vi "replace plot - plot ref - V2.vi"(0 "Plot ref in":refnum<vi>, 1 "Array X IN":dbl[](array[numeric]), 2 "Array Y IN":dbl[](array[numeric]), 3 "text":string="x", 5 "plot index":i32, 6 "cursor action":T2=enum."write", 7 "label":enum16{"hide", "show x", "show y", "show (x,y)"}(ring), 12 "Color Box":u32(colorbox)=327424, 13 "cursor state":T3=enum."boring") -> (14 "Plot ref out":refnum<vi>, 15 "Array X":dbl[](array[numeric]), 16 "Array Y":dbl[](array[numeric]), 19 "2Dwindow bounds out":T1={"min y"=0.0021014740628288917, "max x"=44850.89441339177, "min x"=2.5658109925320947, "max y"=17480.201988350764} {"max y" format="%#9_9f"; "min x" format="%#9_9f"; "max x" format="%#9_9f"})   [LabVIEW 2021]
uses:
  cursor sate.ctl
  cursor action.ctl
  2Dwindow-bounds.ctl
  stack action -- control.ctl
  range multiplier action.ctl
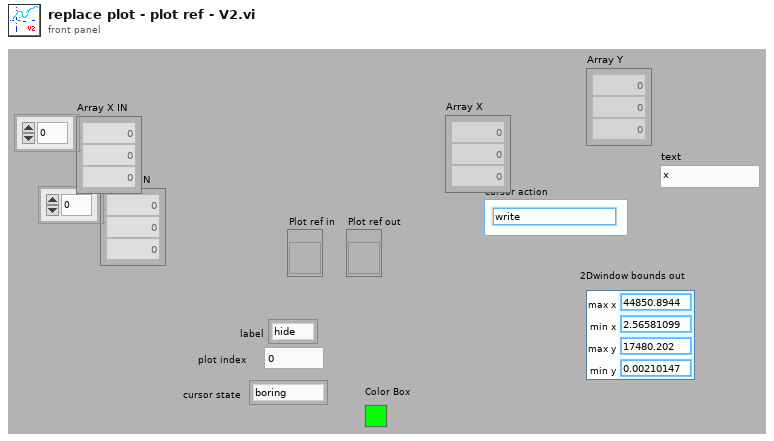
[diagram p1: front panel]
types:
  T1 = typedef "2Dwindow-bounds.ctl" = cluster{"min y":dbl, "max x":dbl, "min x":dbl, "max y":dbl}
  T2 = typedef "cursor action.ctl" = enum16{"range", "read", "write", "check", "zoom out", "smart zoom out", "zoom to aspect ratio 1", "zoom to win", "zoom out 20%", "zoom in 20%", "-empty", "smart zoom out&aspect", "move range left 20%", "move range right 20%", "move range up 20%", "move range down 20%", "zoom to X win", "zoom to Y win", "zoom out X", "zoom out Y", "zoom in X", "zoom in Y", "check plot scale", "set plot color", "set Xlabel", "set Ylabel", "set cursor color"}
  T3 = typedef "cursor sate.ctl" = enum16{"normal", "alert", "fuzzy", "interesting", "boring", "colored"}
  T4 = typedef "stack action -- control.ctl" = enum16{"push", "pop", "check", "init"}
  T5 = typedef "range multiplier action.ctl" = enum16{"shift", "zoom", "check"}
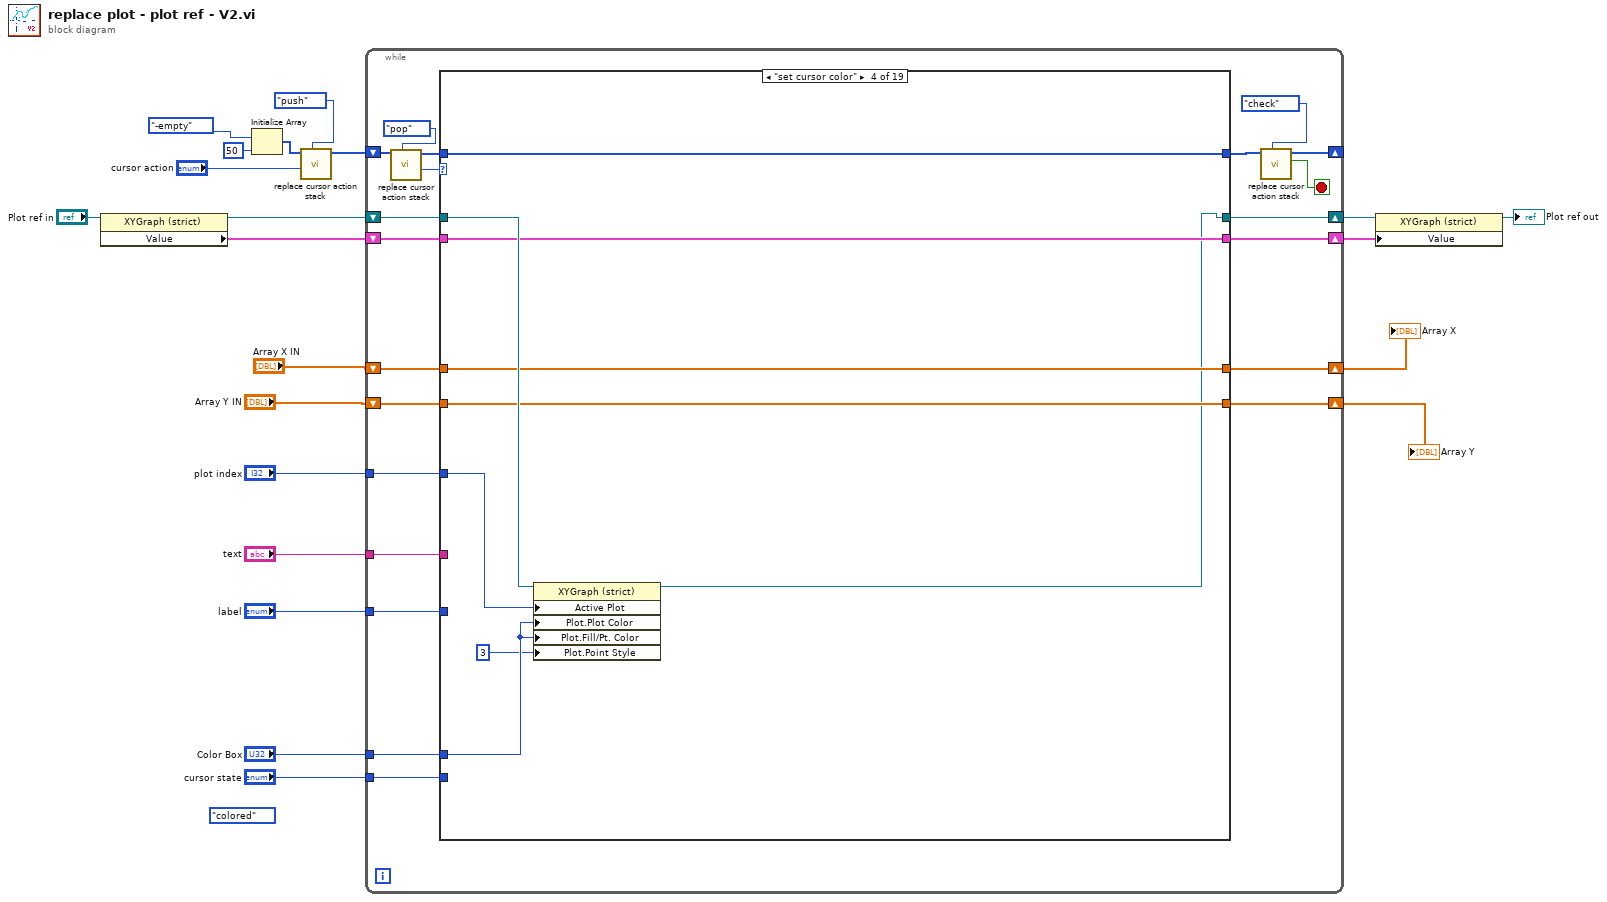
[diagram p0: block diagram]
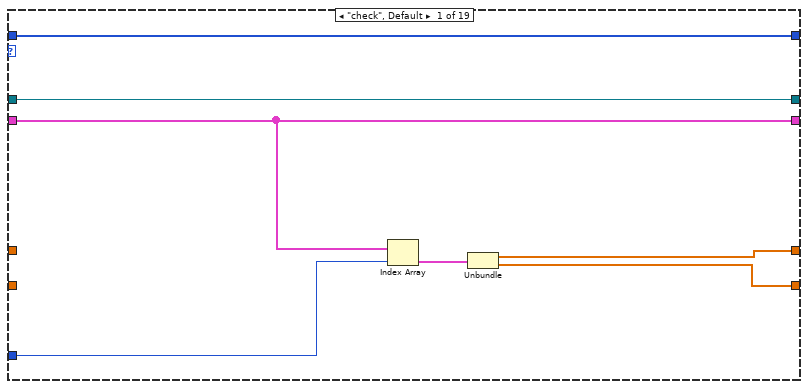
[diagram p2: hidden frame]
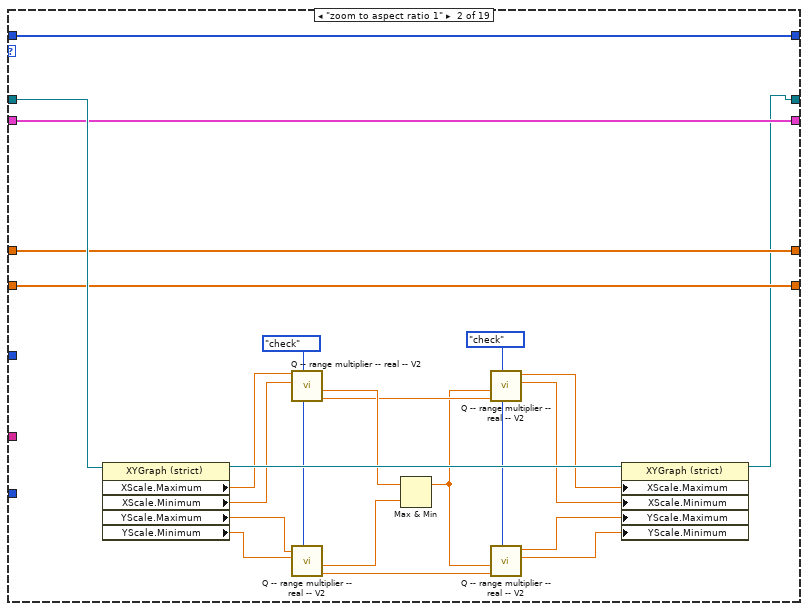
[diagram p3: hidden frame]
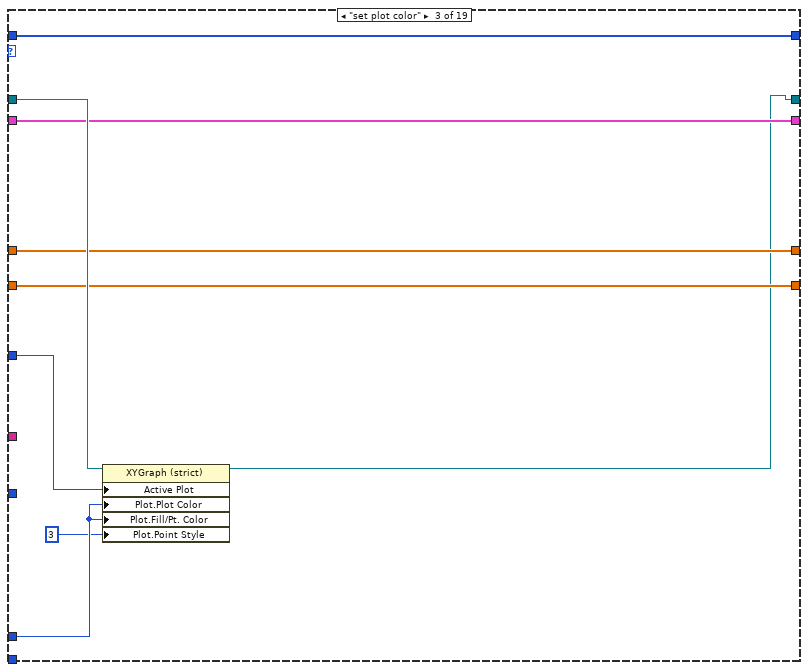
[diagram p4: hidden frame]
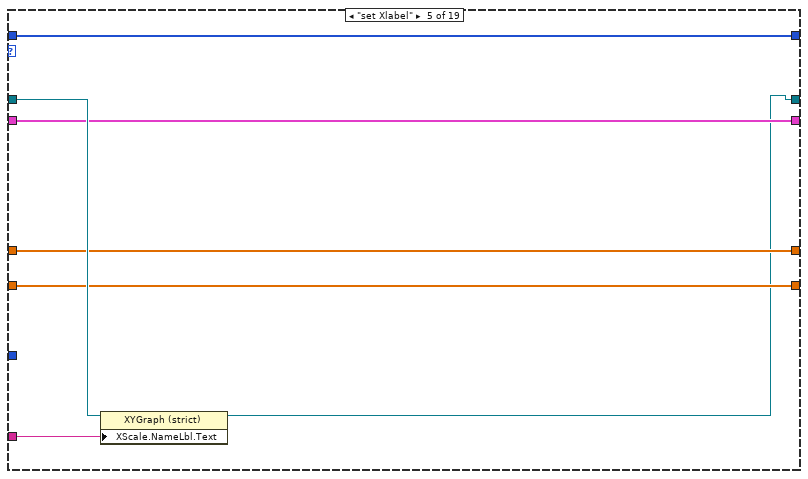
[diagram p5: hidden frame]
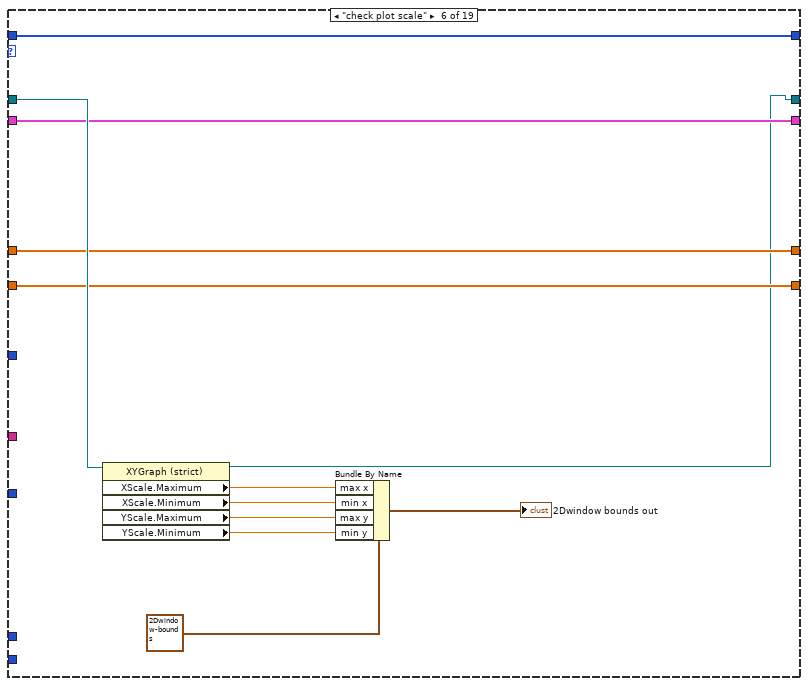
[diagram p6: hidden frame]
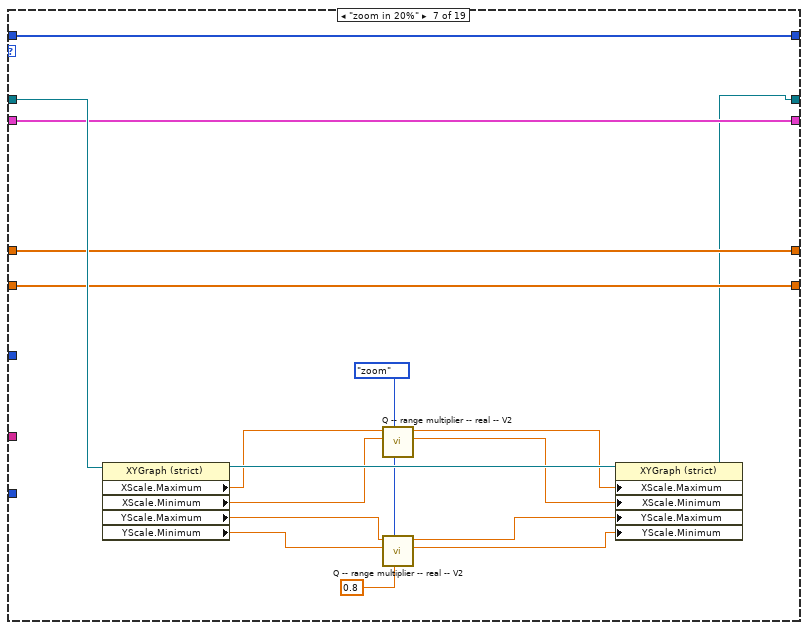
[diagram p7: hidden frame]
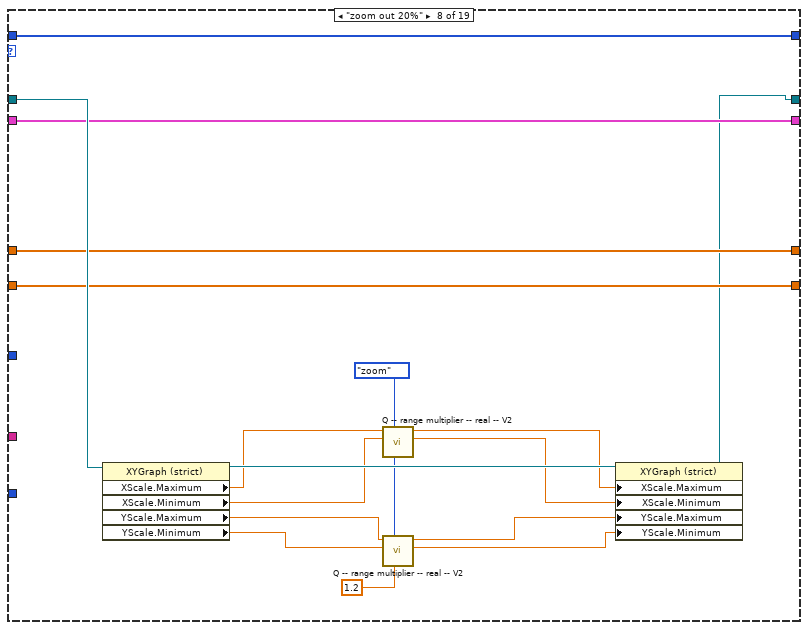
[diagram p8: hidden frame]
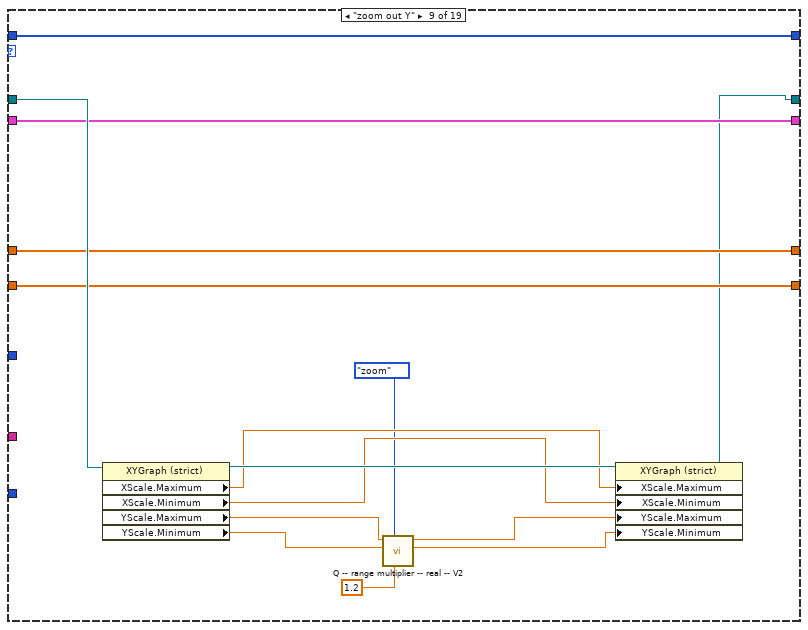
[diagram p9: hidden frame]
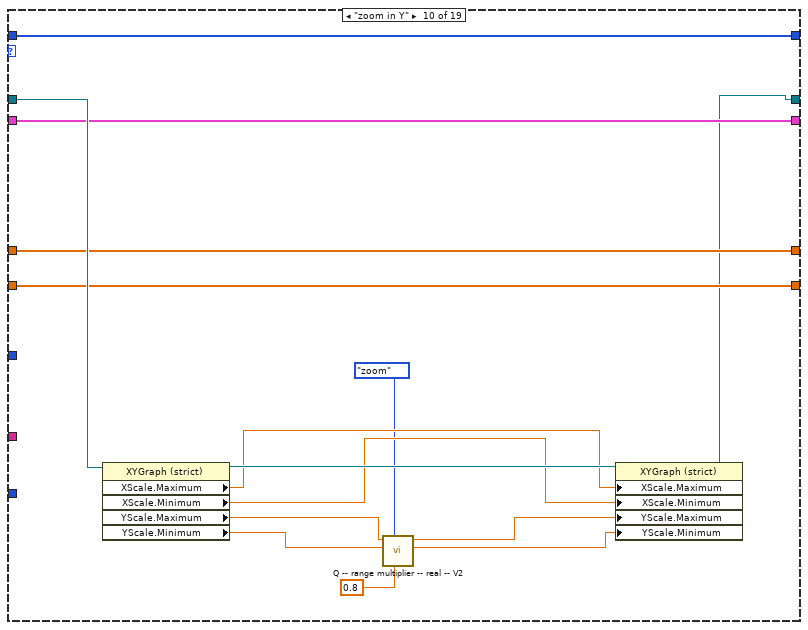
[diagram p10: hidden frame]
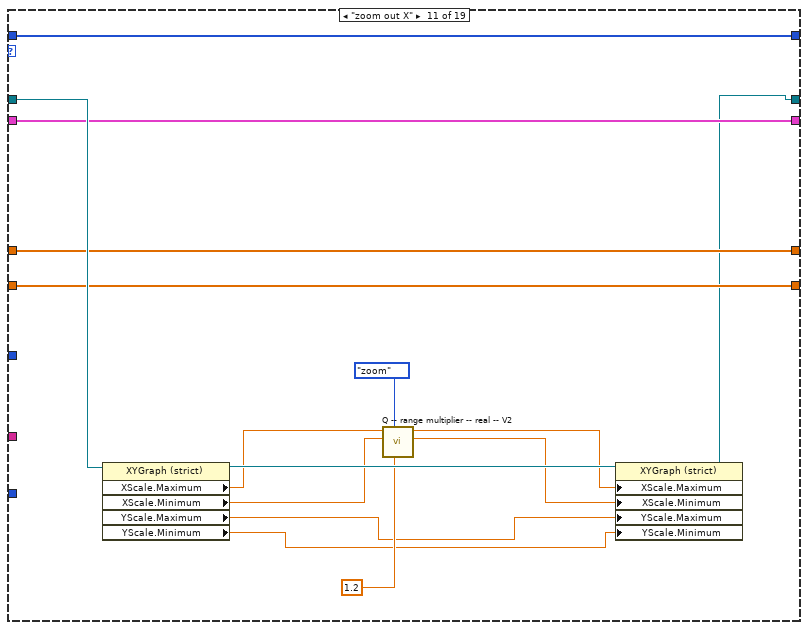
[diagram p11: hidden frame]
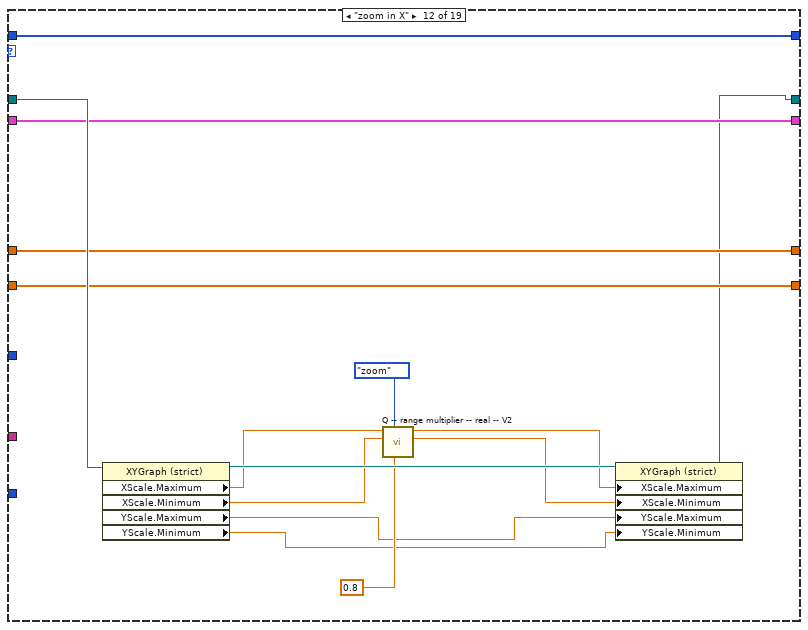
[diagram p12: hidden frame]
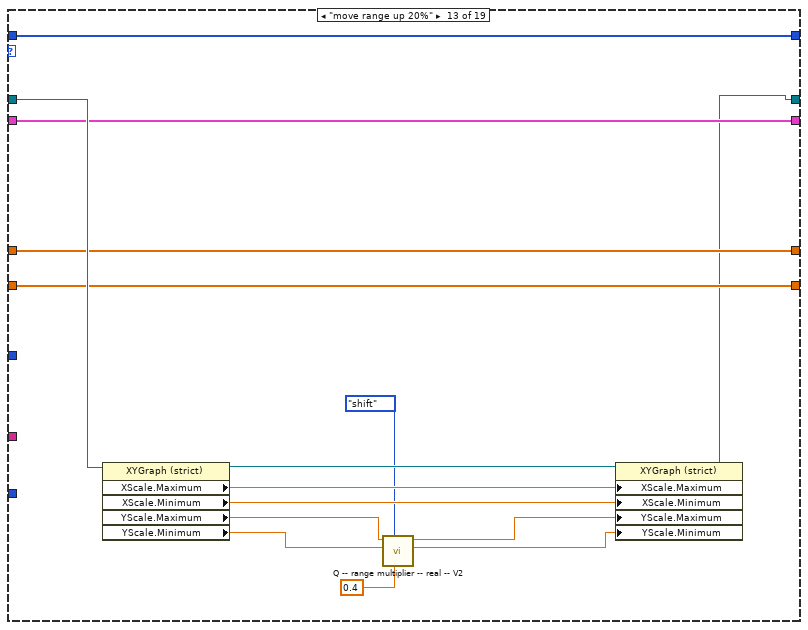
[diagram p13: hidden frame]
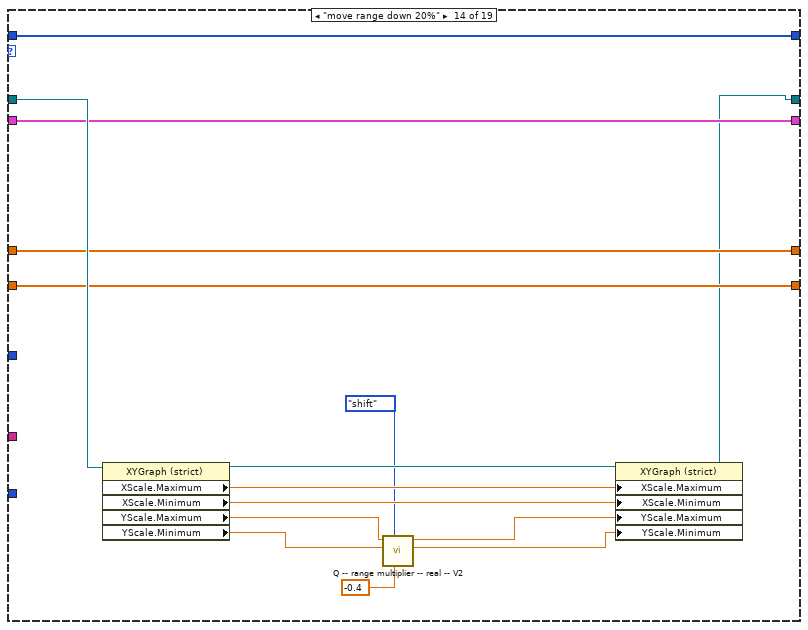
[diagram p14: hidden frame]
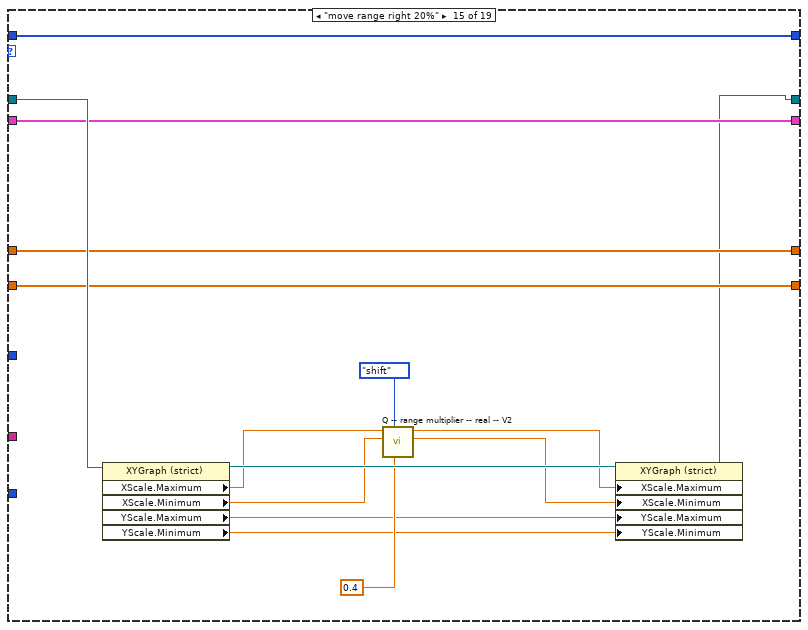
[diagram p15: hidden frame]
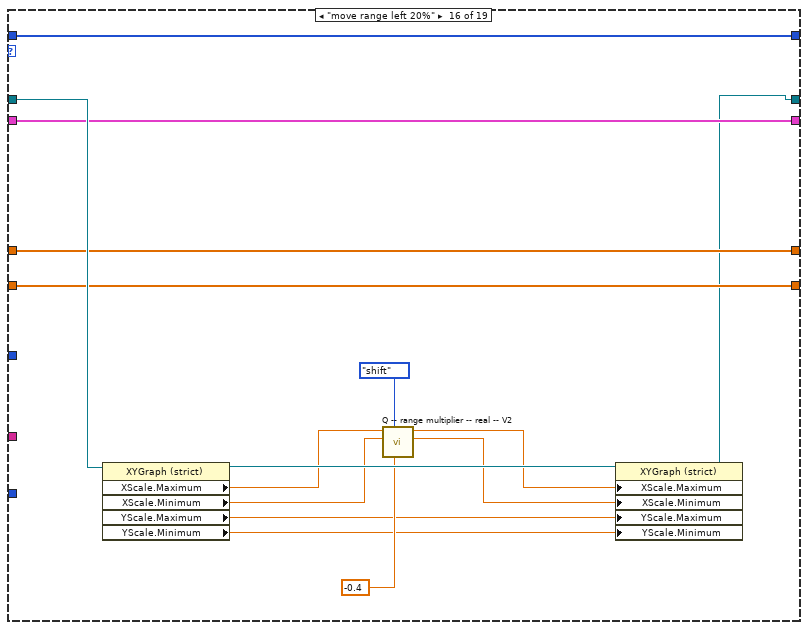
[diagram p16: hidden frame]
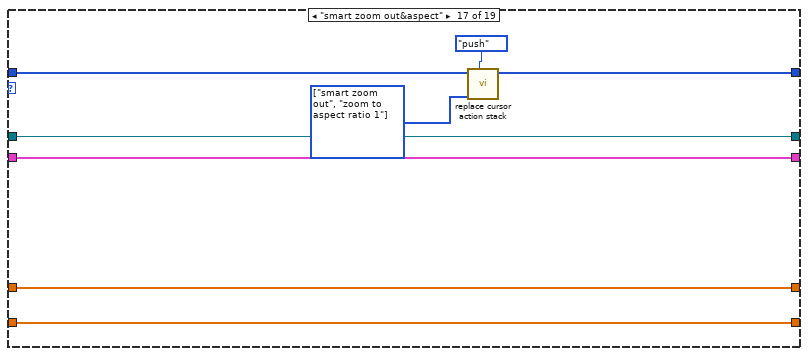
[diagram p17: hidden frame]
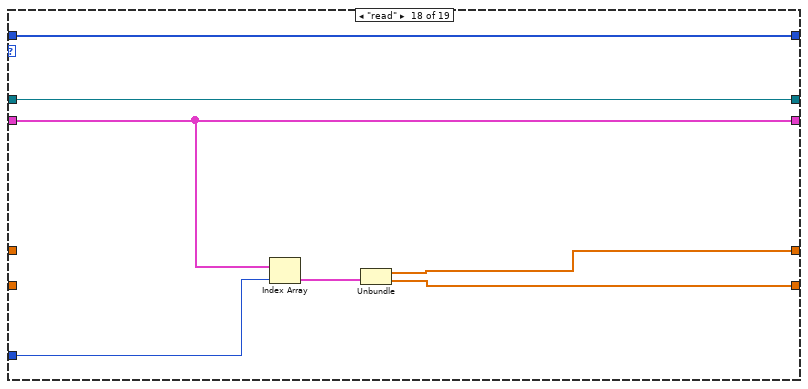
[diagram p18: hidden frame]
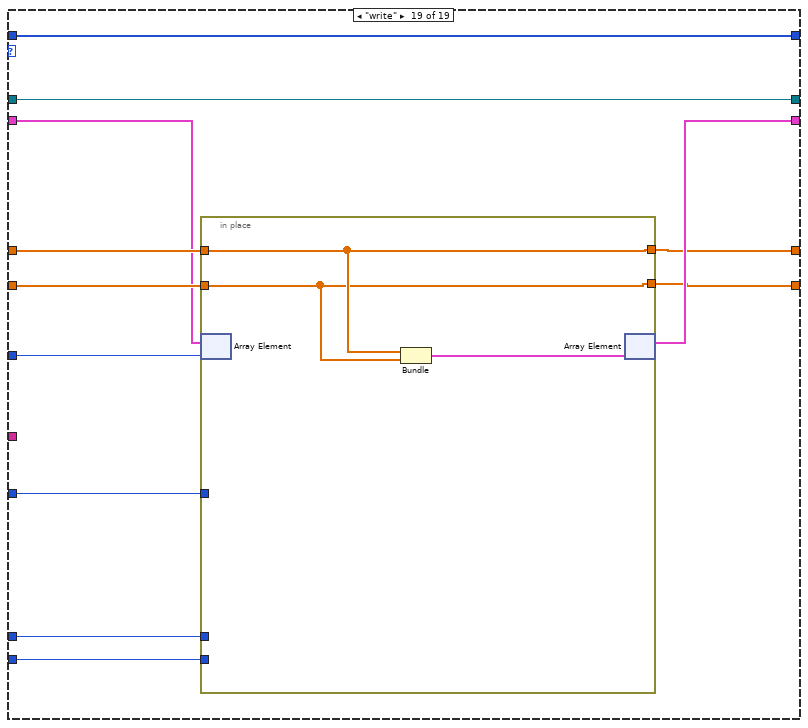
[diagram p19: hidden frame]
diagram:
  (unwired) cursor_sate."colored" ("cursor state")
  n1 = property on="Property Node" class="XYGraph (strict)"(reference="Plot ref in") -> (reference out=w13:refnum<vi>, "Value"=w20:cluster{dbl[], dbl[]}[])  [unwired: 1 in, 1 out]
  n2 = Initialize Array(cursor_action."-empty" ("cursor action"), 50 ("dimension size")) -> (w9:T2[])
  n3 = call "replace cursor action stack.vi"("stack action"=stack_action_--_control."push", "cursor action"="cursor action", "command stack In"=w9) -> ("command stack Out"=w6:T2[])  [unwired: 6 in, 2 out]
  n4 = while {
    tunnel: "plot index" -> [w42]
    tunnel: "label" -> [w38]
    tunnel: "Color Box" -> [w37]
    tunnel: "cursor state" -> [w36]
    shift-right: [w33] -> w12
    shift-left: w20 -> [w39]
    shift-right: [w35] -> w14
    shift-left: w13 -> [w34]
    shift-right: [w28] -> _
    shift-left: w6 -> [w32]
    shift-right: [w25] -> w4
    shift-left: "Array Y IN" -> [w41]
    shift-right: [w24] -> w5
    shift-left: "Array X IN" -> [w40]
    tunnel: "text" -> [w22]
    stop <- w29 stop-if-true
    n5 = call "replace cursor action stack.vi"("stack action"=stack_action_--_control."pop", "command stack In"=w32) -> ("cursor action Out"=w30:T2, "command stack Out"=w26:T2[])  [unwired: 7 in, 1 out]
    n6 = case shown="\"set cursor color\"" w30 {
      tunnel: w42 -> [w47 _ w75 w84 _ _ _ _ _ _ _ _ _ _ _ _ _ w277 w285]
      tunnel: w39 -> [w48 w69 w79 w88 w95 w107 w123 w140 w155 w170 w185 w200 w215 w230 w245 w260 w263 w276 w287]
      tunnel: w41 -> [_ w67 w77 w86 w93 w105 w121 w138 w153 w168 w183 w198 w213 w228 w243 w258 w265 _ w288]
      tunnel: w40 -> [_ w68 w78 w87 w94 w106 w122 w139 w154 w169 w184 w199 w214 w229 w244 w259 w266 _ w289]
      tunnel: [w44 w68 w78 w87 w94 w106 w122 w139 w154 w169 w184 w199 w214 w229 w244 w259 w266 w272 w284] -> w24
      tunnel: [w43 w67 w77 w86 w93 w105 w121 w138 w153 w168 w183 w198 w213 w228 w243 w258 w265 w271 w283] -> w25
      tunnel: w38 -> [_ _ _ _ _ _ _ _ _ _ _ _ _ _ _ _ _ _ w282]
      tunnel: w37 -> [_ _ w73 w82 _ _ _ _ _ _ _ _ _ _ _ _ _ _ w281]
      tunnel: w36 -> [_ _ _ _ _ _ _ _ _ _ _ _ _ _ _ _ _ _ w280]
      tunnel: [w49 w65 w74 w83 w91 w103 w119 w136 w151 w166 w181 w196 w211 w226 w241 w256 w264 w275 w279] -> w35
      tunnel: w34 -> [w49 w70 w80 w89 w96 w108 w124 w141 w156 w171 w186 w201 w216 w231 w246 w261 w264 w275 w279]
      tunnel: [w48 w69 w79 w88 w95 w107 w123 w140 w155 w170 w185 w200 w215 w230 w245 w260 w263 w276 w286] -> w33
      tunnel: [w46 w66 w76 w85 w92 w104 w120 w137 w152 w167 w182 w197 w212 w227 w242 w257 w268 w274 w278] -> w27
      tunnel: w26 -> [w46 w66 w76 w85 w92 w104 w120 w137 w152 w167 w182 w197 w212 w227 w242 w257 w269 w274 w278]
      tunnel: w22 -> [_ _ _ _ w90 _ _ _ _ _ _ _ _ _ _ _ _ _ _]
      frame "check", Default {
        n7 = Index Array(array=w48, index=w47) -> (element=w45:cluster{dbl[], dbl[]})
        n8 = Unbundle(w45) -> (w44:dbl[], w43:dbl[])
      }
      frame "zoom to aspect ratio 1" {
        w54 = range_multiplier_action."check" ("rage multiplier action")
        w60 = range_multiplier_action."check" ("rage multiplier action")
        n9 = property on="Property Node" class="XYGraph (strict)"(reference=w70) -> (reference out=w71:refnum<vi>, "XScale.Maximum"=w64:dbl, "XScale.Minimum"=w63:dbl, "YScale.Maximum"=w62:dbl, "YScale.Minimum"=w61:dbl)  [unwired: 1 in, 1 out]
        n10 = call "Q -- range multiplier -- real -- V2.vi"("rage multiplier action"=w60, "lower"=w63, "upper"=w64) -> ("center OUT"=w57:dbl, "window OUT"=w59:dbl)  [unwired: 5 in, 2 out]
        n11 = call "Q -- range multiplier -- real -- V2.vi"("rage multiplier action"=w60, "lower"=w61, "upper"=w62) -> ("center OUT"=w56:dbl, "window OUT"=w58:dbl)  [unwired: 5 in, 2 out]
        n12 = Max & Min(x=w59, y=w58) -> (max(x,y)=w55:dbl)  [unwired: 1 out]
        n13 = call "Q -- range multiplier -- real -- V2.vi"("rage multiplier action"=w54, "center"=w57, "window"=w55) -> ("lower OUT"=w50:dbl, "upper OUT"=w51:dbl)  [unwired: 5 in, 2 out]
        n14 = call "Q -- range multiplier -- real -- V2.vi"("rage multiplier action"=w54, "center"=w56, "window"=w55) -> ("lower OUT"=w52:dbl, "upper OUT"=w53:dbl)  [unwired: 5 in, 2 out]
        n15 = property on="Property Node" class="XYGraph (strict)"(reference=w71, "XScale.Maximum"=w51, "XScale.Minimum"=w50, "YScale.Maximum"=w53, "YScale.Minimum"=w52) -> (reference out=w65:refnum<vi>)  [unwired: 1 in, 1 out]
      }
      frame "set plot color" {
        n16 = property on="Property Node" class="XYGraph (strict)"(reference=w80, "Active Plot"=w75, "Plot.Plot Color"=w73, "Plot.Fill/Pt. Color"=w73, "Plot.Point Style"=u8 3) -> (reference out=w74:refnum<vi>)  [unwired: 1 in, 1 out]
      }
      frame "set cursor color" {
        n17 = property on="Property Node" class="XYGraph (strict)"(reference=w89, "Active Plot"=w84, "Plot.Plot Color"=w82, "Plot.Fill/Pt. Color"=w82, "Plot.Point Style"=u8 3) -> (reference out=w83:refnum<vi>)  [unwired: 1 in, 1 out]
      }
      frame "set Xlabel" {
        n18 = property on="Property Node" class="XYGraph (strict)"(reference=w96, "XScale.NameLbl.Text"=w90) -> (reference out=w91:refnum<vi>)  [unwired: 1 in, 1 out]
      }
      frame "check plot scale" {
        n19 = property on="Property Node" class="XYGraph (strict)"(reference=w108) -> (reference out=w103:refnum<vi>, "XScale.Maximum"=w101:dbl, "XScale.Minimum"=w100:dbl, "YScale.Maximum"=w99:dbl, "YScale.Minimum"=w98:dbl)  [unwired: 1 in, 1 out]
        n20 = Bundle By Name(cluster=T1 {"min y"=0.0021014740628288917, "max x"=44850.89441339177, "min x"=2.5658109925320947, "max y"=17480.201988350764} ("2Dwindow bounds out"), "max x"=w101, "min x"=w100, "max y"=w99, "min y"=w98) -> (→"2Dwindow bounds out":T1)
      }
      frame "zoom in 20%" {
        w110 = range_multiplier_action."zoom" ("rage multiplier action")
        w109 = 0.8
        n21 = property on="Property Node" class="XYGraph (strict)"(reference=w124) -> (reference out=w125:refnum<vi>, "XScale.Maximum"=w118:dbl, "XScale.Minimum"=w117:dbl, "YScale.Maximum"=w114:dbl, "YScale.Minimum"=w113:dbl)  [unwired: 1 in, 1 out]
        n22 = call "Q -- range multiplier -- real -- V2.vi"("factor"=w109, "rage multiplier action"=w110, "lower"=w117, "upper"=w118) -> ("lower OUT"=w115:dbl, "upper OUT"=w116:dbl)  [unwired: 4 in, 2 out]
        n23 = call "Q -- range multiplier -- real -- V2.vi"("factor"=w109, "rage multiplier action"=w110, "lower"=w113, "upper"=w114) -> ("lower OUT"=w111:dbl, "upper OUT"=w112:dbl)  [unwired: 4 in, 2 out]
        n24 = property on="Property Node" class="XYGraph (strict)"(reference=w125, "XScale.Maximum"=w116, "XScale.Minimum"=w115, "YScale.Maximum"=w112, "YScale.Minimum"=w111) -> (reference out=w119:refnum<vi>)  [unwired: 1 in, 1 out]
      }
      frame "zoom out 20%" {
        w127 = range_multiplier_action."zoom" ("rage multiplier action")
        w126 = 1.2
        n25 = property on="Property Node" class="XYGraph (strict)"(reference=w141) -> (reference out=w142:refnum<vi>, "XScale.Maximum"=w135:dbl, "XScale.Minimum"=w134:dbl, "YScale.Maximum"=w131:dbl, "YScale.Minimum"=w130:dbl)  [unwired: 1 in, 1 out]
        n26 = call "Q -- range multiplier -- real -- V2.vi"("factor"=w126, "rage multiplier action"=w127, "lower"=w134, "upper"=w135) -> ("lower OUT"=w132:dbl, "upper OUT"=w133:dbl)  [unwired: 4 in, 2 out]
        n27 = call "Q -- range multiplier -- real -- V2.vi"("factor"=w126, "rage multiplier action"=w127, "lower"=w130, "upper"=w131) -> ("lower OUT"=w128:dbl, "upper OUT"=w129:dbl)  [unwired: 4 in, 2 out]
        n28 = property on="Property Node" class="XYGraph (strict)"(reference=w142, "XScale.Maximum"=w133, "XScale.Minimum"=w132, "YScale.Maximum"=w129, "YScale.Minimum"=w128) -> (reference out=w136:refnum<vi>)  [unwired: 1 in, 1 out]
      }
      frame "zoom out Y" {
        n29 = property on="Property Node" class="XYGraph (strict)"(reference=w156) -> (reference out=w157:refnum<vi>, "XScale.Maximum"=w145:dbl, "XScale.Minimum"=w144:dbl, "YScale.Maximum"=w150:dbl, "YScale.Minimum"=w149:dbl)  [unwired: 1 in, 1 out]
        n30 = call "Q -- range multiplier -- real -- V2.vi"("factor"=1.2, "rage multiplier action"=range_multiplier_action."zoom", "lower"=w149, "upper"=w150) -> ("lower OUT"=w147:dbl, "upper OUT"=w148:dbl)  [unwired: 4 in, 2 out]
        n31 = property on="Property Node" class="XYGraph (strict)"(reference=w157, "XScale.Maximum"=w145, "XScale.Minimum"=w144, "YScale.Maximum"=w148, "YScale.Minimum"=w147) -> (reference out=w151:refnum<vi>)  [unwired: 1 in, 1 out]
      }
      frame "zoom in Y" {
        n32 = property on="Property Node" class="XYGraph (strict)"(reference=w171) -> (reference out=w172:refnum<vi>, "XScale.Maximum"=w160:dbl, "XScale.Minimum"=w159:dbl, "YScale.Maximum"=w165:dbl, "YScale.Minimum"=w164:dbl)  [unwired: 1 in, 1 out]
        n33 = call "Q -- range multiplier -- real -- V2.vi"("factor"=0.8, "rage multiplier action"=range_multiplier_action."zoom", "lower"=w164, "upper"=w165) -> ("lower OUT"=w162:dbl, "upper OUT"=w163:dbl)  [unwired: 4 in, 2 out]
        n34 = property on="Property Node" class="XYGraph (strict)"(reference=w172, "XScale.Maximum"=w160, "XScale.Minimum"=w159, "YScale.Maximum"=w163, "YScale.Minimum"=w162) -> (reference out=w166:refnum<vi>)  [unwired: 1 in, 1 out]
      }
      frame "zoom out X" {
        n35 = property on="Property Node" class="XYGraph (strict)"(reference=w186) -> (reference out=w187:refnum<vi>, "XScale.Maximum"=w180:dbl, "XScale.Minimum"=w179:dbl, "YScale.Maximum"=w174:dbl, "YScale.Minimum"=w173:dbl)  [unwired: 1 in, 1 out]
        n36 = call "Q -- range multiplier -- real -- V2.vi"("factor"=1.2, "rage multiplier action"=range_multiplier_action."zoom", "lower"=w179, "upper"=w180) -> ("lower OUT"=w177:dbl, "upper OUT"=w178:dbl)  [unwired: 4 in, 2 out]
        n37 = property on="Property Node" class="XYGraph (strict)"(reference=w187, "XScale.Maximum"=w178, "XScale.Minimum"=w177, "YScale.Maximum"=w174, "YScale.Minimum"=w173) -> (reference out=w181:refnum<vi>)  [unwired: 1 in, 1 out]
      }
      frame "zoom in X" {
        n38 = property on="Property Node" class="XYGraph (strict)"(reference=w201) -> (reference out=w202:refnum<vi>, "XScale.Maximum"=w195:dbl, "XScale.Minimum"=w194:dbl, "YScale.Maximum"=w189:dbl, "YScale.Minimum"=w188:dbl)  [unwired: 1 in, 1 out]
        n39 = call "Q -- range multiplier -- real -- V2.vi"("factor"=0.8, "rage multiplier action"=range_multiplier_action."zoom", "lower"=w194, "upper"=w195) -> ("lower OUT"=w192:dbl, "upper OUT"=w193:dbl)  [unwired: 4 in, 2 out]
        n40 = property on="Property Node" class="XYGraph (strict)"(reference=w202, "XScale.Maximum"=w193, "XScale.Minimum"=w192, "YScale.Maximum"=w189, "YScale.Minimum"=w188) -> (reference out=w196:refnum<vi>)  [unwired: 1 in, 1 out]
      }
      frame "move range up 20%" {
        n41 = property on="Property Node" class="XYGraph (strict)"(reference=w216) -> (reference out=w217:refnum<vi>, "XScale.Maximum"=w204:dbl, "XScale.Minimum"=w205:dbl, "YScale.Maximum"=w210:dbl, "YScale.Minimum"=w209:dbl)  [unwired: 1 in, 1 out]
        n42 = call "Q -- range multiplier -- real -- V2.vi"("factor"=0.4, "rage multiplier action"=range_multiplier_action."shift", "lower"=w209, "upper"=w210) -> ("lower OUT"=w207:dbl, "upper OUT"=w208:dbl)  [unwired: 4 in, 2 out]
        n43 = property on="Property Node" class="XYGraph (strict)"(reference=w217, "XScale.Maximum"=w204, "XScale.Minimum"=w205, "YScale.Maximum"=w208, "YScale.Minimum"=w207) -> (reference out=w211:refnum<vi>)  [unwired: 1 in, 1 out]
      }
      frame "move range down 20%" {
        n44 = property on="Property Node" class="XYGraph (strict)"(reference=w231) -> (reference out=w232:refnum<vi>, "XScale.Maximum"=w219:dbl, "XScale.Minimum"=w220:dbl, "YScale.Maximum"=w225:dbl, "YScale.Minimum"=w224:dbl)  [unwired: 1 in, 1 out]
        n45 = call "Q -- range multiplier -- real -- V2.vi"("factor"=-0.4, "rage multiplier action"=range_multiplier_action."shift", "lower"=w224, "upper"=w225) -> ("lower OUT"=w222:dbl, "upper OUT"=w223:dbl)  [unwired: 4 in, 2 out]
        n46 = property on="Property Node" class="XYGraph (strict)"(reference=w232, "XScale.Maximum"=w219, "XScale.Minimum"=w220, "YScale.Maximum"=w223, "YScale.Minimum"=w222) -> (reference out=w226:refnum<vi>)  [unwired: 1 in, 1 out]
      }
      frame "move range right 20%" {
        n47 = property on="Property Node" class="XYGraph (strict)"(reference=w246) -> (reference out=w247:refnum<vi>, "XScale.Maximum"=w240:dbl, "XScale.Minimum"=w239:dbl, "YScale.Maximum"=w234:dbl, "YScale.Minimum"=w233:dbl)  [unwired: 1 in, 1 out]
        n48 = call "Q -- range multiplier -- real -- V2.vi"("factor"=0.4, "rage multiplier action"=range_multiplier_action."shift", "lower"=w239, "upper"=w240) -> ("lower OUT"=w237:dbl, "upper OUT"=w238:dbl)  [unwired: 4 in, 2 out]
        n49 = property on="Property Node" class="XYGraph (strict)"(reference=w247, "XScale.Maximum"=w238, "XScale.Minimum"=w237, "YScale.Maximum"=w234, "YScale.Minimum"=w233) -> (reference out=w241:refnum<vi>)  [unwired: 1 in, 1 out]
      }
      frame "move range left 20%" {
        n50 = property on="Property Node" class="XYGraph (strict)"(reference=w261) -> (reference out=w262:refnum<vi>, "XScale.Maximum"=w255:dbl, "XScale.Minimum"=w254:dbl, "YScale.Maximum"=w249:dbl, "YScale.Minimum"=w248:dbl)  [unwired: 1 in, 1 out]
        n51 = call "Q -- range multiplier -- real -- V2.vi"("factor"=-0.4, "rage multiplier action"=range_multiplier_action."shift", "lower"=w254, "upper"=w255) -> ("lower OUT"=w252:dbl, "upper OUT"=w253:dbl)  [unwired: 4 in, 2 out]
        n52 = property on="Property Node" class="XYGraph (strict)"(reference=w262, "XScale.Maximum"=w253, "XScale.Minimum"=w252, "YScale.Maximum"=w249, "YScale.Minimum"=w248) -> (reference out=w256:refnum<vi>)  [unwired: 1 in, 1 out]
      }
      frame "smart zoom out&aspect" {
        w267 = T2[] [enum."smart zoom out", enum."zoom to aspect ratio 1"] items=["range", "read", "write", "check", "zoom out", "smart zoom out", "zoom to aspect ratio 1", "zoom to win", "zoom out 20%", "zoom in 20%", "-empty", "smart zoom out&aspect", "move range left 20%", "move range right 20%", "move range up 20%", "move range down 20%", "zoom to X win", "zoom to Y win", "zoom out X", "zoom out Y", "zoom in X", "zoom in Y", "check plot scale", "set plot color", "set Xlabel", "set Ylabel", "set cursor color"] ("action list I")
        n53 = call "replace cursor action stack.vi"("stack action"=stack_action_--_control."push", "action list I"=w267, "command stack In"=w269) -> ("command stack Out"=w268:T2[])  [unwired: 6 in, 2 out]
      }
      frame "read" {
        n54 = Index Array(array=w276, index=w277) -> (element=w273:cluster{dbl[], dbl[]})
        n55 = Unbundle(w273) -> (w272:dbl[], w271:dbl[])
      }
      frame "write" {
        n56 = in-place {
          in-place-border: w289 -> [w292]
          in-place-border: w288 -> [w291]
          in-place-border: [w292] -> w284
          in-place-border: [w291] -> w283
          in-place-border: w282 -> [_]
          in-place-border: w281 -> [_]
          in-place-border: w280 -> [_]
          n57 = in-place-array #1(w287, w285) -> ()  [unwired: 1 out]
          n58 = Bundle("Array X IN"=w292, "Array Y IN"=w291) -> (w290:cluster{"Array X IN":dbl[], "Array Y IN":dbl[]})  [unwired: 1 in]
          n59 = in-place-array #1(w290) -> (w286:cluster{dbl[], dbl[]}[])  [unwired: 1 out]
        }
      }
    }
    n60 = call "replace cursor action stack.vi"("stack action"=stack_action_--_control."check", "command stack In"=w27) -> ("stack is empty ?"=w29:bool, "command stack Out"=w28:T2[])  [unwired: 7 in, 1 out]
  }
  "Array X" <- w5
  "Array Y" <- w4
  n61 = property on="Property Node" class="XYGraph (strict)"(reference=w14, "Value"=w12) -> (reference out=→"Plot ref out":refnum<vi>)  [unwired: 1 in, 1 out]
